vi "load control values from file.vi"(8 "error in (no error)":errorcluster, 10 "datalog path (use dialog)":path, 11 "VI ref":refnum<vi>) -> (0 "error out":errorcluster)   [LabVIEW 2013]
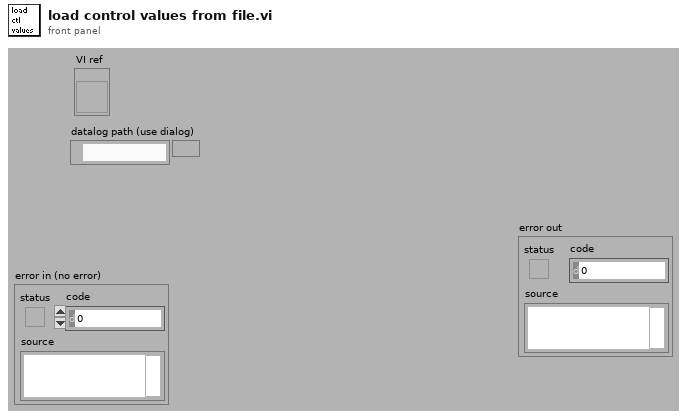
[diagram p1: front panel]
types:
  T1 = enum16{"open", "replace", "create", "open or create", "replace or create", "replace or create with confirmation"}
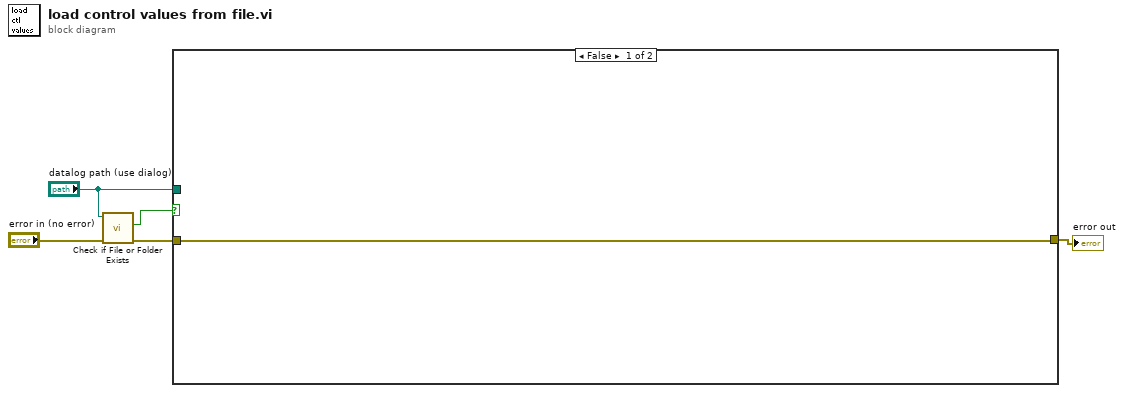
[diagram p0: block diagram]
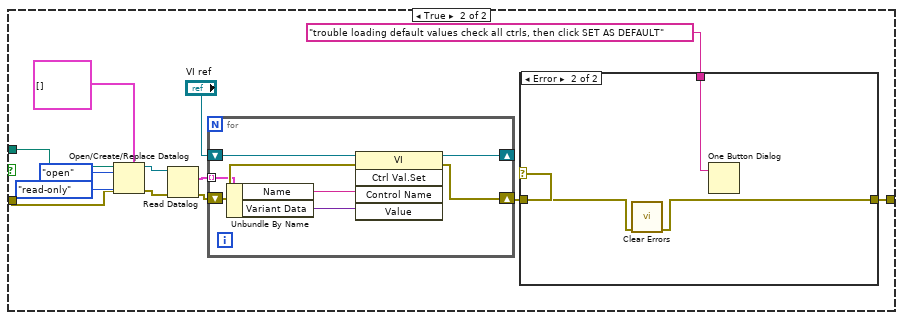
[diagram p2: hidden frame]
diagram:
  n1 = call <vilib>:"Check if File or Folder Exists.vi"("error in (no error)"="error in (no error)", "path"="datalog path (use dialog)") -> ("error out"=w3:errorcluster, "file or folder exists?"=w1:bool)  [unwired: 7 in, 1 out]
  n2 = case shown="False" w1 {
    tunnel: [w6 w10] -> w5
    tunnel: "datalog path (use dialog)" -> [_ w8]
    tunnel: w3 -> [w6 w7]
    frame False {
    }
    frame True {
      n3 = Open/Create/Replace Datalog(5:cluster{"Name":string, "Variant Data":variant}[] [] ("Control Value:Get All [Variant]"), 8:w7, 9:enum16{"read/write", "read-only", "write-only"}."read-only" ("access (0:read/write)"), 10:T1."open" ("operation (0:open)"), 11:w8) -> (0:w17:errorcluster, 3:w16:refnum<k1>)  [unwired: 1 in, 1 out]
      n4 = Read Datalog(4:w17, 7:w16) -> (0:w14:errorcluster, 2:w15:cluster{"Name":string, "Variant Data":variant}[])  [unwired: 1 in, 1 out]
      n5 = for {
        tunnel: w15 -> [w28] mode=indexing
        shift-right: [w25] -> w11
        shift-left: w14 -> [w29]
        shift-right: [w24] -> _
        shift-left: "VI ref" -> [w30]
        n6 = Unbundle By Name(w28) -> ("Name"=w27:string, "Variant Data"=w26:variant)
        n7 = invoke class="VI" method="Ctrl Val.Set"(reference=w30, error in=w29, "Control Name"=w27, "Value"=w26) -> (reference out=w24:refnum<vi>, error out=w25:errorcluster)  [unwired: 1 in, 3 out]
      }
      n8 = case shown="Error" w11 {
        tunnel: w11 -> [w20 w22]
        tunnel: [w20 w21] -> w10
        tunnel: "trouble loading default values check all ctrls, then click SET AS DEFAULT" ("message") -> [_ w23]
        frame No Error {
        }
        frame Error {
          n9 = call <vilib>:"Clear Errors.vi"("error in (no error)"=w22) -> ("error out"=w21:errorcluster)  [unwired: 6 in]
          n10 = One Button Dialog(message=w23) -> ()  [unwired: 1 in, 1 out]
        }
      }
    }
  }
  "error out" <- w5
